vi "speed ro zero.vi"() -> (3 "output cluster":T1)   [LabVIEW 2015]
uses:
  PC/QMH Fundamentals - Message Cluster.ctl
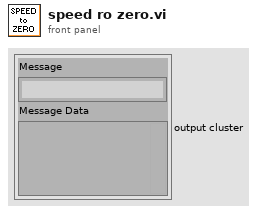
[diagram p1: front panel]
types:
  T1 = typedef "QMH Fundamentals - Message Cluster.ctl" = cluster{"Message":string, "Message Data":variant}
  T2 = cluster{"identifier":u32, "extended?":bool, "type":u8, "payload":u8[]}[]
  T3 = cluster{"Data":cluster{"date/time string":string, "array of cans":cluster{"identifier":u32, "extended?":bool, "type":u8, "payload":u8[]}[]}, "bool":bool}
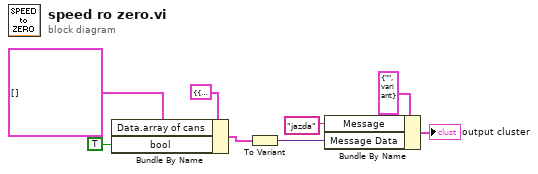
[diagram p0: block diagram]
diagram:
  n1 = Bundle By Name(cluster=T3 {"Data"={"date/time string"="", "array of cans"=[]}, "bool"=TRUE} ("jazda"), "Data.array of cans"=T2 [], "bool"=TRUE) -> (w5:T3)
  n2 = To Variant(anything=w5) -> (Variant=w1:variant)
  n3 = Bundle By Name(cluster=T1 {"Message"="", "Message Data"=variant} ("Message Cluster"), "Message"="jazda", "Message Data"=w1) -> (→"output cluster":T1)
